vi "Goto Wavelength.vi"(8 "error in (no error)":errorcluster, 10 "Target WL":dbl, 11 "Spectrometer iHR320.lvclass In":refnum<class "Spectrometer iHR320.lvclass">) -> (0 "error out":errorcluster, 2 "Actual WL":dbl, 3 "Spectrometer iHR320.lvclass Out":refnum<class "Spectrometer iHR320.lvclass">)   [LabVIEW 2009, in "Spectrometer iHR320.lvclass"]
doc: "Closes the slits, moves to the target wavelength, then restores the slits."
uses:
  Spectrometer iHR320.lvclass
  Spectrometer iHR320.lvclass/Spectrometer iHR320.ctl
panel:
  out "Exit Slit Width":dbl
  out "Front Slit Width":dbl
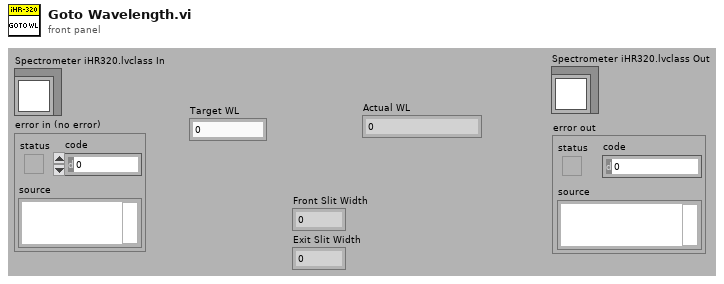
[diagram p1: front panel]
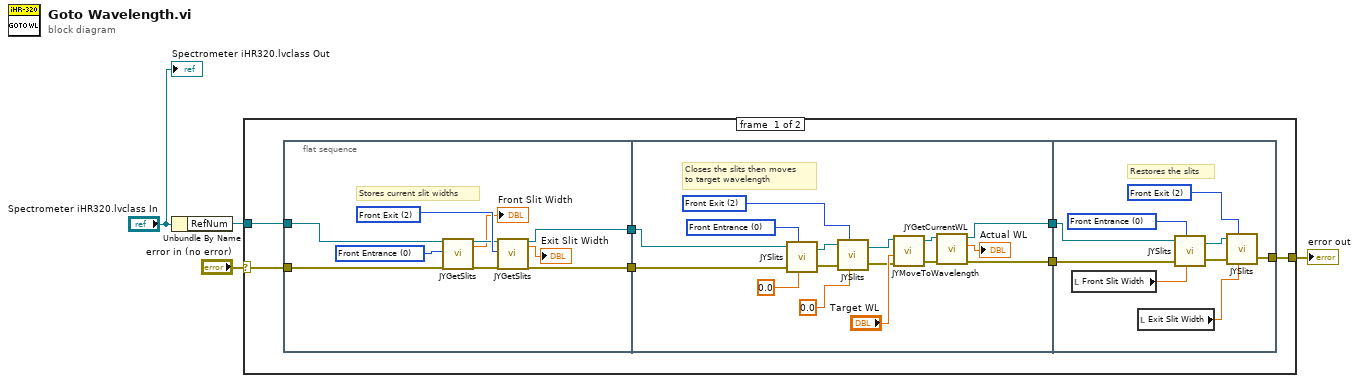
[diagram p0: block diagram]
diagram:
  n1 = Unbundle By Name("Spectrometer iHR320.lvclass In") -> ("RefNum"=w4:refnum<k7>)
  n2 = case shown="No Error" "error in (no error)" {
    selector: "error in (no error)" -> [w11 w47]
    tunnel: w4 -> [w10 _]
    tunnel: [w5 w47] -> w1
    frame #0 {
      n3 = flat-sequence {
        tunnel: w11 -> [w19]
        tunnel: w10 -> [w16]
        tunnel: [w17] -> w9
        tunnel: [w14] -> w8
        tunnel: w9 -> [w24]
        tunnel: w8 -> [w25]
        tunnel: [w23] -> w7
        tunnel: [w22] -> w6
        tunnel: w7 -> [w40]
        tunnel: w6 -> [w39]
        tunnel: [w38] -> w5
        frame #0 {
          w20 = u16 2 items=["Front Entrance", "Side Entrance", "Front Exit", "Side Exit", "First Intermediate", "Second Intermediate"] ("Slit")
          w21 = u16 0 items=["Front Entrance", "Side Entrance", "Front Exit", "Side Exit", "First Intermediate", "Second Intermediate"] ("Slit")
          # "Stores current slit widths"
          n4 = call "JYGetSlits.vi"("MonoRefNum IN"=w16, "Slit"=w21, "error in (no error)"=w19) -> ("MonoRefNum Out"=w15:refnum<k7>, "Slit Width"=→"Front Slit Width":dbl, "error out"=w18:errorcluster)  [unwired: 13 in, 1 out]
          n5 = call "JYGetSlits.vi"("MonoRefNum IN"=w15, "Slit"=w20, "error in (no error)"=w18) -> ("MonoRefNum Out"=w14:refnum<k7>, "Slit Width"=→"Exit Slit Width":dbl, "error out"=w17:errorcluster)  [unwired: 13 in, 1 out]
        }
        frame #1 {
          w28 = u16 2 items=["Front Entrance", "Side Entrance", "Front Exit", "Side Exit", "First Intermediate", "Second Intermediate"] ("Slit")
          w26 = u16 0 items=["Front Entrance", "Side Entrance", "Front Exit", "Side Exit", "First Intermediate", "Second Intermediate"] ("Slit")
          # "Closes the slits then moves\nto target wavelength"
          n6 = call "JYSlits.vi"("JYMONOLib.IJYMonoReqd In"=w25, "Slit"=w26, "error in (no error)"=w24, "Slit Width"=0.0) -> ("JYMONOLib.IJYMonoReqd Out"=w30:refnum<k7>, "error out"=w31:errorcluster)  [unwired: 1 in]
          n7 = call "JYSlits.vi"("JYMONOLib.IJYMonoReqd In"=w30, "Slit"=w28, "error in (no error)"=w31, "Slit Width"=0.0) -> ("JYMONOLib.IJYMonoReqd Out"=w32:refnum<k7>, "error out"=w33:errorcluster)  [unwired: 1 in]
          n8 = call "JYMoveToWavelength.vi"("error in (no error)"=w33, "Target WL"="Target WL", "RefNum In"=w32) -> ("error out"=w36:errorcluster, "Refnum Out"=w35:refnum<k7>)  [unwired: 1 in, 1 out]
          n9 = call "JYGetCurrentWL.vi"("error in (no error)"=w36, "JYMONOLib.IJYMonoReqd In"=w35) -> ("error out"=w23:errorcluster, "Current WL"=→"Actual WL":dbl, "JYMONOLib.IJYMonoReqd Out"=w22:refnum<k7>)  [unwired: 6 in, 1 out]
        }
        frame #2 {
          w43 = u16 2 items=["Front Entrance", "Side Entrance", "Front Exit", "Side Exit", "First Intermediate", "Second Intermediate"] ("Slit")
          w42 = u16 0 items=["Front Entrance", "Side Entrance", "Front Exit", "Side Exit", "First Intermediate", "Second Intermediate"] ("Slit")
          # "Restores the slits"
          n10 = local read "Front Slit Width"() -> (w41:dbl)
          n11 = local read "Exit Slit Width"() -> (w46:dbl)
          n12 = call "JYSlits.vi"("JYMONOLib.IJYMonoReqd In"=w39, "Slit"=w42, "error in (no error)"=w40, "Slit Width"=w41) -> ("JYMONOLib.IJYMonoReqd Out"=w44:refnum<k7>, "error out"=w45:errorcluster)  [unwired: 1 in]
          n13 = call "JYSlits.vi"("JYMONOLib.IJYMonoReqd In"=w44, "Slit"=w43, "error in (no error)"=w45, "Slit Width"=w46) -> ("error out"=w38:errorcluster)  [unwired: 1 in, 1 out]
        }
      }
    }
    frame #1 {
    }
  }
  "error out" <- w1
  "Spectrometer iHR320.lvclass Out" <- "Spectrometer iHR320.lvclass In"
